vi "Delete Items.vi"(6 "indent":i32, 8 "error in (no error)":errorcluster, 9 "Copy? (F)":bool, 10 "Indices to remove":i32[](array[numeric]), 11 "BetterBoxHandle in":refnum<class "BetterBoxHandle.lvclass">) -> (0 "error out":errorcluster, 2 "items removed":refnum<class "BetterItem.lvclass">[](array[class]), 3 "BetterBoxHandle out":refnum<class "BetterBoxHandle.lvclass">)   [LabVIEW 2020, in "BetterDragAndDrop.lvlib" / "BetterBoxHandle.lvclass"]
uses:
  BetterBoxHandle.lvclass
  C:/DSCE code/Open-source/betterdraganddrop_GIT/Source/Classes/BetterHandle/BetterHandle.lvclass
  BetterTreeItem/BetterItem.lvclass
  BetterHandle/BetterHandle.lvclass/BetterHandle.ctl
  7d65aa2f-1078-45c8-b733-894fd3ad821d.vi
  BetterHandle/BetterHandle.lvclass
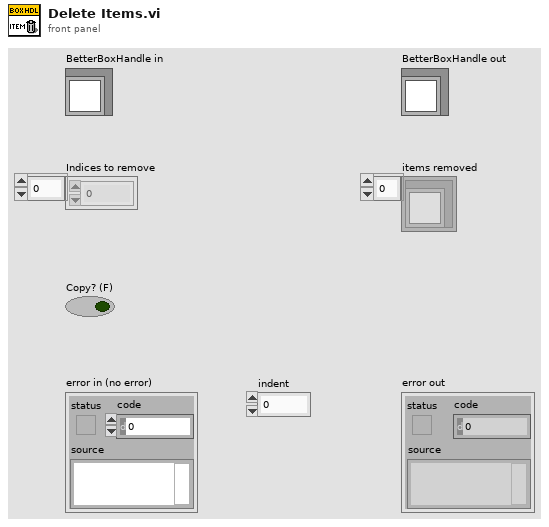
[diagram p1: front panel]
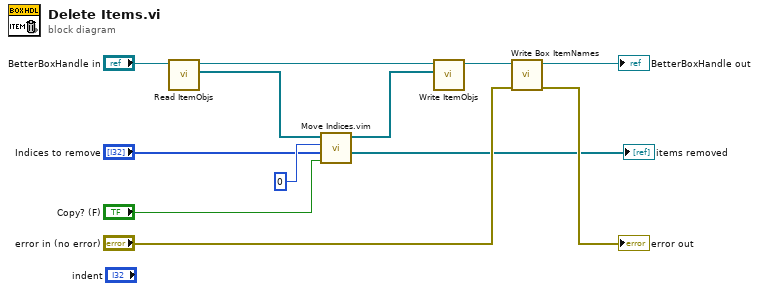
[diagram p0: block diagram]
diagram:
  n1 = call "Read ItemObjs.vi"("BetterHandle in"="BetterBoxHandle in") -> ("ItemObjs"=w10:refnum<class "BetterItem.lvclass">[], "BetterHandle out"=w8:refnum<class "BetterBoxHandle.lvclass">)  [unwired: 9 in]
  n2 = call "Move Indices.vim"("Copy?"="Copy? (F)", "Indices to move"="Indices to remove", "insertion index"=0, "Array"=w10) -> ("elements to be inserted"=→"items removed":refnum<class "BetterItem.lvclass">[], "modified array"=w7:refnum<class "BetterItem.lvclass">[])  [unwired: 5 in, 1 out]
  n3 = call "Write ItemObjs.vi"("ItemObjs"=w7, "BetterHandle in"=w8) -> ("BetterHandle out"=w6:refnum<class "BetterBoxHandle.lvclass">)  [unwired: 9 in]
  n4 = call-dynamic "Write Box ItemNames.vi"("error in (no error)"="error in (no error)", "BetterBoxHandle in"=w6) -> ("error out"=→"error out":errorcluster, "BetterBoxHandle out"=→"BetterBoxHandle out":refnum<class "BetterBoxHandle.lvclass">)  [unwired: 8 in]
